vi "Conv1D_Top.vi"() -> ()   [LabVIEW 2020]
doc: "This benchmark is designed to demonstrate execution performance improvement when executing FFT and IFFT operations on a GPU."
uses:
  <vilib>/Analysis/baseanly.llb/Mean (DBL).vi
  <vilib>/Analysis/1siggen.llb/Ramp Pattern by Delta.vi
  <vilib>/Utility/file.llb/Read Delimited Spreadsheet (DBL).vi
  <vilib>/Ngene/CuLab - GPU Accelerated Toolkit/Toolkit/CuLab.lvlib
  <vilib>/Analysis/NI_AALBase.lvlib
panel:
  in  "CPU Iteration":i32=3
  out "CuLab Mean Performance Gain":dbl[](array[numeric])=[1.0, 21.15550240134334, 2.150127019247679] format="%#.2g"
  out "Releative Exec Time vs CuLab (smaller is better)":cluster{i32[], "all rows":dbl[]}[](graph)=[{[32, 64, 128, 256, 512, 1024, 2048, 4096, 8192, 16384, 32768, 65536, 131072, 262144, 524288, 1048576, 2097152, 4194304, 8388608], "all rows"=[1.0, 1.0, 1.0, 1.0, 1.0, 1.0, 1.0, 1.0, 1.0, 1.0, 1.0, 1.0, 1.0, 1.0, 1.0, 1.0, 1.0, 1.0, 1.0]}, {[32, 64, 128, 256, 512, 1024, 2048, 4096, 8192, 16384, 32768, 65536, 131072, 262144, 524288, 1048576, 2097152, 4194304, 8388608], "all rows"=[0.01756007317582555, 0.016584334182935315, 0.025495751584069883, 0.046109510605750074, 0.08436639174537595, 0.19503816763949391, 0.3126022890031592, 0.6247258769756535, 1.2544094062732074, 2.7816419531963863, 5.753390257987012, 14.351283238045562, 23.17681161598989, 30.63054892919567, 40.34997783118421, 48.787817534178686, 69.9424732892676, 78.75487582579176, 84.84883334950125]}, {[32, 64, 128, 256, 512, 1024, 2048, 4096, 8192, 16384, 32768, 65536, 131072, 262144, 524288, 1048576, 2097152, 4194304, 8388608], "all rows"=[3.0383549015381206, 2.44248411598812, 2.3905807341105567, 2.454250719420757, 2.346763090589481, 3.2312977152776625, 2.3404255246144743, 2.2494517533354674, 2.2247461202747876, 2.454389959580728, 2.187845304768891, 2.112282311398667, 1.8762681175877451, 1.8483293557616274, 1.525262224523902, 1.4566653830991367, 1.5601556676397683, 1.5581714895677652, 1.554688876628257]}]
  in  "CuPy CSV":path=path "D:/Ngene/GitHub/culab_examples/Benchmarks/CuPy/results/GeForce_RTX_2080_Ti/Conv1D_CuPy.csv"
  out "Execution Time":cluster{i32[], "all rows":dbl[]}[](graph)=[{[32, 64, 128, 256, 512, 1024, 2048, 4096, 8192, 16384, 32768, 65536, 131072, 262144, 524288, 1048576, 2097152, 4194304, 8388608], "all rows"=[0.00010819999988598283, 0.00014170000031299423, 0.00014120000014372636, 0.0001388000000588363, 0.00014519999967887998, 0.00013099999978294363, 0.0001833000005717622, 0.0001824000000851811, 0.00018710000040300656, 0.0001754000004439149, 0.00019909999991796212, 0.0002181999998356332, 0.00027599999975791434, 0.00041899999996530823, 0.0006769000001440872, 0.001558800000566407, 0.0024154000002454268, 0.0048760999998194166, 0.009647300000324321]}, {[32, 64, 128, 256, 512, 1024, 2048, 4096, 8192, 16384, 32768, 65536, 131072, 262144, 524288, 1048576, 2097152, 4194304, 8388608], "all rows"=[1.8999999156221747e-06, 2.350000158912735e-06, 3.600000127335079e-06, 6.4000000747910235e-06, 1.2250000054336851e-05, 2.5549999918439426e-05, 5.729999975301325e-05, 0.00011395000001357403, 0.00023470000041925232, 0.0004878999998254585, 0.001145499999893218, 0.0031314500001826673, 0.006396800000402436, 0.012834200000270357, 0.027312899999742513, 0.0760504499999115, 0.1689390500000627, 0.38401664999992136, 0.8185621500001616]}, {[32, 64, 128, 256, 512, 1024, 2048, 4096, 8192, 16384, 32768, 65536, 131072, 262144, 524288, 1048576, 2097152, 4194304, 8388608], "all rows"=[0.00032875000000000005, 0.0003461, 0.00033755000000000005, 0.00034065000000000007, 0.00034075, 0.00042330000000000004, 0.000429, 0.0004103, 0.00041625000000000006, 0.0004305, 0.0004356, 0.00046090000000000004, 0.00051785, 0.0007744500000000001, 0.00103245, 0.00227065, 0.0037684000000000003, 0.0075978, 0.014998550000000001]}]
  out "GPU Model":string="NVIDIA GeForce RTX 2080 Ti"
  out "CPU Model":string="Intel(R) Core(TM) i7-8700K"
  in  "GPU Iteration":i32=200
  in  "Size Stop(2^n)":i32=23
  in  "Size Start(2^n)":i32=5
  out "Size":i32[](array[numeric])=[32, 64, 128, 256, 512, 1024, 2048, 4096, 8192, 16384, 32768, 65536, 131072, 262144, 524288, 1048576, 2097152, 4194304, 8388608] format="%.2p"
  # "Conv1D Benchmark"
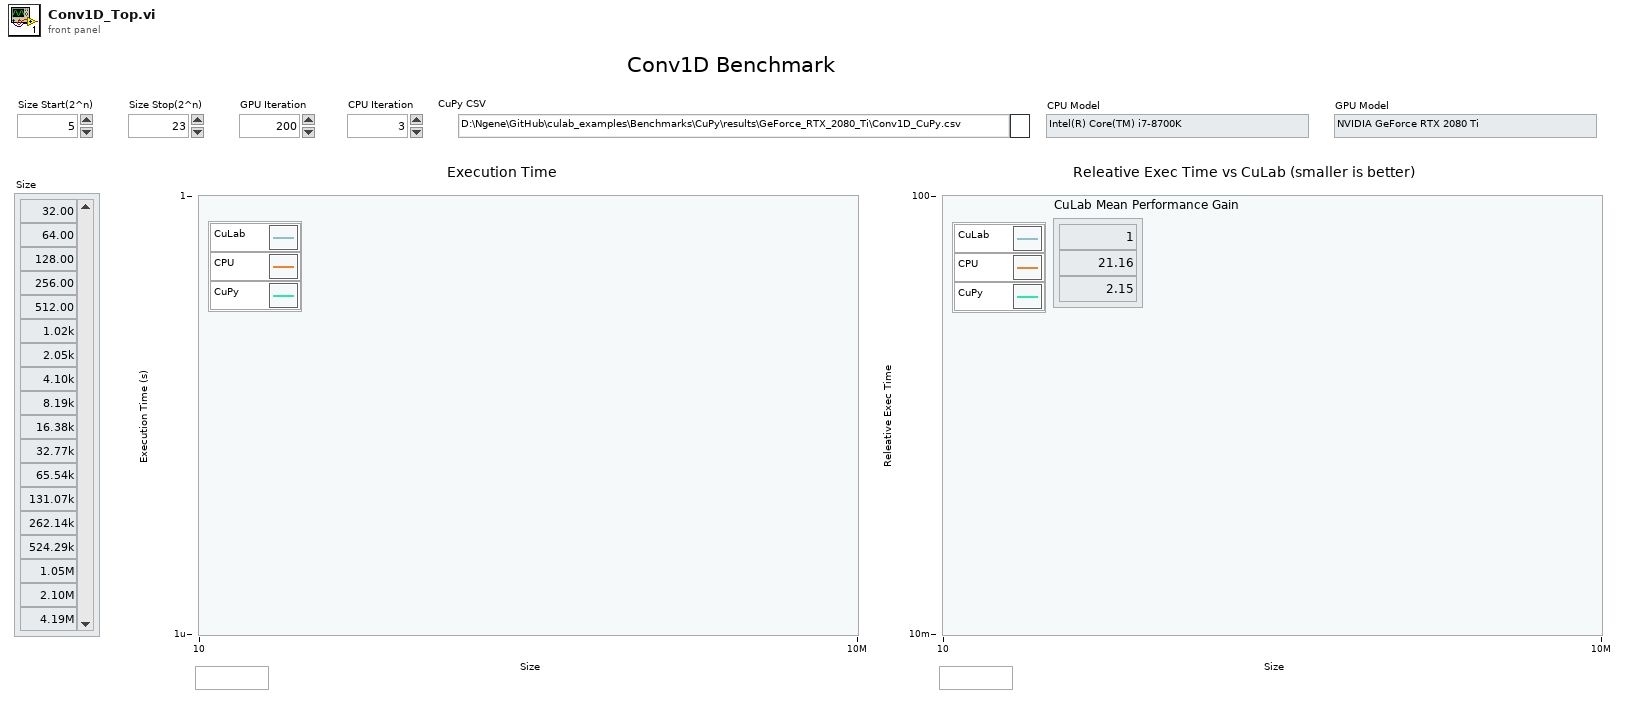
[diagram p1: front panel]
types:
  T1 = typedef "CuLab.lvlib/Properties.ctl" = cluster{"Device ID":i32, "Name":string}
  T2 = typedef "imagedata.ctl" = cluster{"image type":i32, "image depth":i32, "image":u8[], "mask":u8[], "colors":u32[], "Rectangle":cluster{"left":i16, "top":i16, "right":i16, "bottom":i16}}
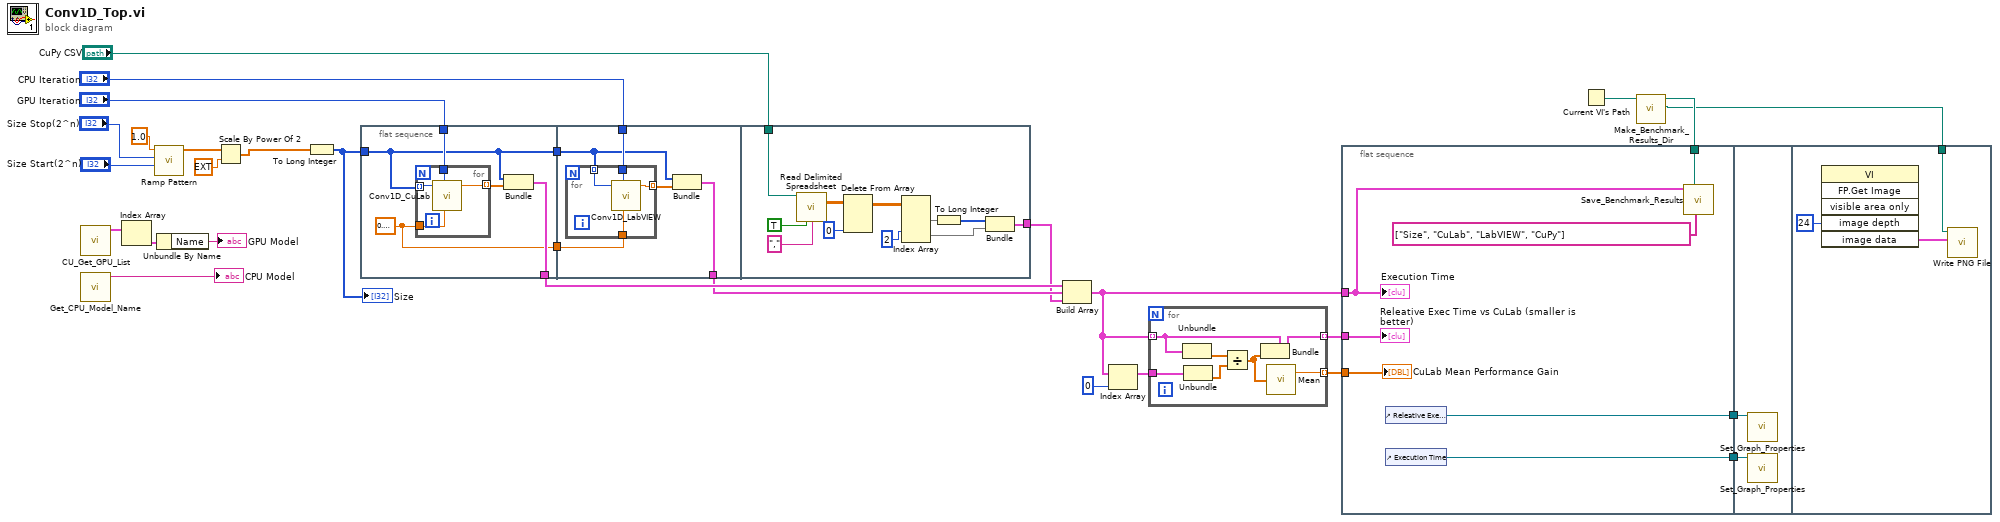
[diagram p0: block diagram]
diagram:
  n1 = call <vilib>:"CU_Get_GPU_List.vi"() -> ("Devices"=w28:T1[])  [unwired: 10 in, 1 out]
  n2 = call "Get_CPU_Model_Name.vi"() -> ("CPU Model"=→"CPU Model":string)  [unwired: 11 in]
  n3 = Index Array(array=w28) -> (element=w27:T1)  [unwired: 1 in]
  n4 = call-poly <vilib>:"Ramp Pattern.vi"("start"="Size Start(2^n)", "end"="Size Stop(2^n)", "delta"=1.0) -> ("Ramp Pattern"=w10:dbl[])  [unwired: 6 in, 2 out]
  n5 = Unbundle By Name(w27) -> ("Name"=→"GPU Model":string)
  n6 = Scale By Power Of 2(n=w10, x=ext 1.0) -> (x*2^n=w12:ext[])
  n7 = To Long Integer(number=w12) -> (32bit integer=w9:i32[])
  "Size" <- w9
  n8 = flat-sequence {
    tunnel: [w31] -> w25
    tunnel: [w32] -> w26
    tunnel: w9 -> [w32]
    tunnel: "GPU Iteration" -> [w34]
    tunnel: [w30] -> w8
    tunnel: w26 -> [w41]
    tunnel: "CPU Iteration" -> [w43]
    tunnel: [w40] -> w23
    tunnel: w8 -> [w39]
    tunnel: "CuPy CSV" -> [w58]
    tunnel: [w50] -> w19
    frame #0 {
      w30 = sgl 0.1 ("Kernel Relative Size")
      n9 = for {
        tunnel: w34 -> [w37]
        tunnel: w32 -> [w38] mode=indexing
        tunnel: [w35] -> w33 mode=indexing
        tunnel: w30 -> [w36]
        n10 = call "Conv1D_CuLab.vi"("Kernel Relative Size"=w36, "No. of Repetition"=w37, "Size"=w38) -> ("Results(s)"=w35:dbl)  [unwired: 8 in]
      }
      n11 = Bundle(w32, w33) -> (w31:cluster{i32[], dbl[]})  [unwired: 1 in]
    }
    frame #1 {
      n12 = for {
        tunnel: w41 -> [w47] mode=indexing
        tunnel: w43 -> [w44]
        tunnel: [w46] -> w42 mode=indexing
        tunnel: w39 -> [w45]
        n13 = call "Conv1D_LabVIEW.vi"("Kernel Relative Size"=w45, "No. of Repetition"=w44, "Size"=w47) -> ("Results(s)"=w46:dbl)  [unwired: 8 in]
      }
      n14 = Bundle(w41, w42) -> (w40:cluster{i32[], dbl[]})  [unwired: 1 in]
    }
    frame #2 {
      n15 = call-poly <vilib>:"Read Delimited Spreadsheet.vi"("file path (dialog if empty)"=w58, "transpose? (F)"=TRUE, "delimiter (\\t)"="," ("delimiter (\\t)")) -> ("all rows"=w56:dbl[][])  [unwired: 7 in, 5 out]
      n16 = Delete From Array(array=w56, index (col)=0 ("disabled index (col)")) -> (array with subset deleted=w54:dbl[][])  [unwired: 2 in, 1 out]
      n17 = Index Array(array=w54, index (row) #2=2 ("disabled index (col)")) -> (element #1=w53:dbl[], element #2=w51:dbl[])  [unwired: 3 in]
      n18 = To Long Integer(number=w53) -> (32bit integer=w52:i32[])
      n19 = Bundle(w52, "all rows"=w51) -> (w50:cluster{i32[], "all rows":dbl[]})  [unwired: 1 in]
    }
  }
  n20 = Build Array(w25, w23, w19) -> (w16:cluster{i32[], "all rows":dbl[]}[])
  n21 = Index Array(array=w16, index=0) -> (element=w22:cluster{i32[], "all rows":dbl[]})
  n22 = for {
    tunnel: w16 -> [w65] mode=indexing
    tunnel: w22 -> [w63]
    tunnel: [w64] -> w18 mode=indexing
    tunnel: [w59] -> w17 mode=indexing
    n23 = Unbundle(w65) -> ("all rows"=w62:dbl[])  [unwired: 1 out]
    n24 = Unbundle(w63) -> ("all rows"=w61:dbl[])  [unwired: 1 out]
    n25 = Divide(x=w62, y=w61) -> (x/y=w60:dbl[])
    n26 = Bundle(cluster=w65, "all rows"=w60) -> (w64:cluster{i32[], "all rows":dbl[]})  [unwired: 1 in]
    n27 = call-poly <vilib>:"Mean.vi"("X"=w60) -> ("mean"=w59:dbl)  [unwired: 1 out]
  }
  n28 = flat-sequence {
    tunnel: w18 -> [w72]
    tunnel: w17 -> [w71]
    tunnel: w16 -> [w68]
    tunnel: w4 -> [w69]
    tunnel: [w67] -> w2
    tunnel: [w66] -> w1
    tunnel: w2 -> [w74]
    tunnel: w1 -> [w73]
    tunnel: w3 -> [w76]
    frame #0 {
      n29 = control-ref of="Releative Exec Time vs CuLab (smaller is better)"() -> (w67:refnum<vi>)
      n30 = control-ref of="Execution Time"() -> (w66:refnum<vi>)
      n31 = call "Save_Benchmark_Results.vi"("Header"=string[] ["Size", "CuLab", "LabVIEW", "CuPy"], "file path (dialog if empty)"=w69, "Execution Time"=w68) -> ()  [unwired: 9 in]
      "Execution Time" <- w68
      "CuLab Mean Performance Gain" <- w71
      "Releative Exec Time vs CuLab (smaller is better)" <- w72
    }
    frame #1 {
      n32 = call "Set_Graph_Properties.vi"("Graph"=w74) -> ()  [unwired: 11 in]
      n33 = call "Set_Graph_Properties.vi"("Graph"=w73) -> ()  [unwired: 11 in]
    }
    frame #2 {
      n34 = invoke class="VI" method="FP.Get Image"("image depth"=24 ("Image Depth")) -> ("image data"=w77:T2)  [unwired: 5 in, 5 out]
      n35 = call <vilib>:"Write PNG File.vi"("image data"=w77, "path to PNG file"=w76) -> ()  [unwired: 8 in, 2 out]
    }
  }
  n36 = Current VI's Path() -> (path=w5:path)
  n37 = call "Make_Benchmark_Results_Dir.vi"("Caller Path"=w5) -> ("Caller FP Image Path"=w3:path, "CSV_File"=w4:path)  [unwired: 9 in]
